vi "Read Status (SubVI).vi"(3 "error out 2":errorcluster, 4 "String":string, 5 "String 2":string, 6 "VISA resource name out 2":refnum<visa-resource-name>) -> (0 "error out":errorcluster, 1 "read buffer":string, 2 "VISA resource name out":refnum<visa-resource-name>)   [LabVIEW 2020]
panel:
  out "return count":u32
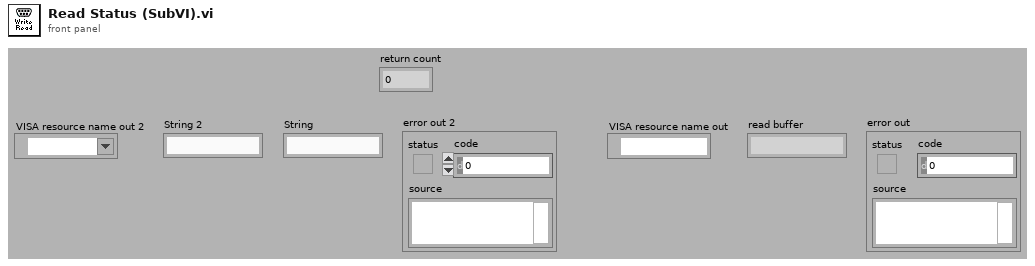
[diagram p1: front panel]
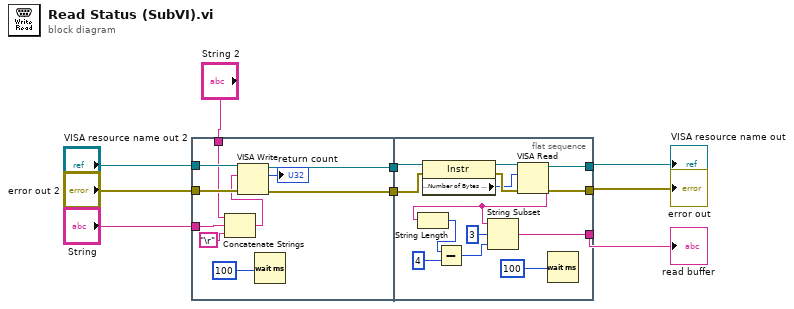
[diagram p0: block diagram]
diagram:
  n1 = flat-sequence {
    tunnel: "VISA resource name out 2" -> [w19]
    tunnel: "error out 2" -> [w18]
    tunnel: "String 2" -> [w17]
    tunnel: "String" -> [w16]
    tunnel: [w14] -> w9
    tunnel: [w13] -> w8
    tunnel: w9 -> [w33]
    tunnel: w8 -> [w32]
    tunnel: [w28] -> w5
    tunnel: [w27] -> w6
    tunnel: [w21] -> w7
    frame #0 {
      n2 = Concatenate Strings(w17, w16, "\r") -> (w15:string)
      n3 = VISA Write(VISA resource name=w19, write buffer=w15, error in (no error)=w18) -> (VISA resource name out=w14:refnum<visa-resource-name>, return count=→"return count":u32, error out=w13:errorcluster)
      n4 = Wait (ms)(milliseconds to wait=u32 100) -> ()  [unwired: 1 out]
    }
    frame #1 {
      n5 = property class="Instr"(reference=w33, error in=w32) -> (reference out=w31:refnum<visa-resource-name>, error out=w30:errorcluster, "Serial Settings:Number of Bytes at Serial Port"=w29:u32)
      n6 = VISA Read(VISA resource name=w31, byte count=w29, error in (no error)=w30) -> (VISA resource name out=w28:refnum<visa-resource-name>, read buffer=w22:string, error out=w27:errorcluster)  [unwired: 1 out]
      n7 = String Length(string=w22) -> (length=w25:i32)
      n8 = Subtract(x=w25, y=4) -> (x-y=w23:i32)
      n9 = String Subset(string=w22, offset (0)=3, length (rest)=w23) -> (substring=w21:string)
      n10 = Wait (ms)(milliseconds to wait=u32 100) -> ()  [unwired: 1 out]
    }
  }
  "read buffer" <- w7
  "error out" <- w6
  "VISA resource name out" <- w5
